vi "fastseq_set_slot-all.vi"(8 "slot":T2 {"slot#" max=4095; "DAC"."DAC offset" min=-1 max=0.5; "DAC"."FastChanNum" max=15 step=1}, 10 "slot number":u16, 11 "FPGA VI Reference In":T1) -> (3 "FPGA VI Reference Out":T1)   [LabVIEW 2013]
uses:
  fpga-bitfile-ref.ctl
  sequence slot/data.ctl
  sequence slot/slot-use.ctl
  sequence slot/triggers.ctl
  sequence slot/DAC.ctl
  sequence slot/DAC_fastseq-offset.ctl
  sequence slot/timing.ctl
  sequence slot/jump.ctl
  sequence slot/slot.xctl
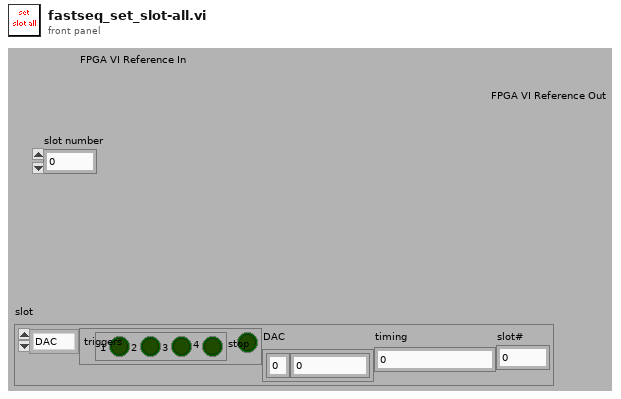
[diagram p1: front panel]
types:
  T1 = typedef "fpga-bitfile-ref.ctl" = refnum<k20>
  T2 = typedef "slot.xctl/data.ctl" = cluster{"use":T3, "Triggers":T4, "DAC":T5, "timing":T7, "slot#":T8}
  T3 = typedef "slot-use.ctl" = enum8{"DAC", "timing", "triggers", "jump"}
  T4 = typedef "triggers.ctl" = cluster{"triggers":cluster{"1":bool, "2":bool, "3":bool, "4":bool}, "stop":bool}
  T5 = typedef "DAC.ctl" = cluster{"FastChanNum":u8, "DAC offset":T6}
  T6 = typedef "DAC_fastseq-offset.ctl" = sgl
  T7 = typedef "timing.ctl" = sgl
  T8 = typedef "jump.ctl" = u16
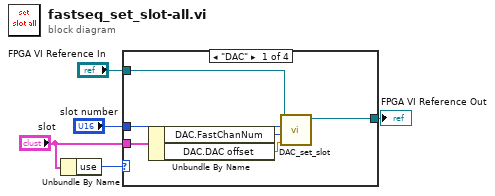
[diagram p0: block diagram]
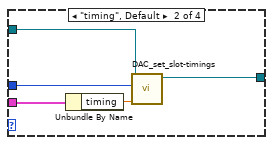
[diagram p2: hidden frame]
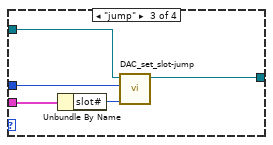
[diagram p3: hidden frame]
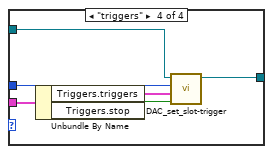
[diagram p4: hidden frame]
diagram:
  n1 = Unbundle By Name("slot") -> ("use"=w3:T3)
  n2 = case shown="\"DAC\"" w3 {
    tunnel: "slot" -> [w11 w16 w21 w27]
    tunnel: "FPGA VI Reference In" -> [w10 w13 w18 w26]
    tunnel: [w9 w12 w19 w25] -> w4
    tunnel: "slot number" -> [w8 w14 w17 w24]
    frame "DAC" {
      n3 = Unbundle By Name(w11) -> ("DAC.FastChanNum"=w7:u8, "DAC.DAC offset"=w6:T6)
      n4 = call "DAC_set_slot.vi"("DAC Offset"=w6, "FastChanNumber"=w7, "slot number"=w8, "FPGA VI Reference In"=w10) -> ("FPGA VI Reference Out"=w9:T1)  [unwired: 7 out]
    }
    frame "timing", Default {
      n5 = Unbundle By Name(w16) -> ("timing"=w15:T7)
      n6 = call "DAC_set_slot-timings.vi"("Time (ms)"=w15, "slot number"=w14, "FPGA VI Reference In"=w13) -> ("FPGA VI Reference Out"=w12:T1)  [unwired: 8 out]
    }
    frame "jump" {
      n7 = Unbundle By Name(w21) -> ("slot#"=w20:T8)
      n8 = call "DAC_set_slot-jump.vi"("JumpTo"=w20, "slot number"=w17, "FPGA VI Reference In"=w18) -> ("FPGA VI Reference Out"=w19:T1)  [unwired: 8 out]
    }
    frame "triggers" {
      n9 = Unbundle By Name(w27) -> ("Triggers.triggers"=w23:cluster{"1":bool, "2":bool, "3":bool, "4":bool}, "Triggers.stop"=w22:bool)
      n10 = call "DAC_set_slot-trigger.vi"("Stop"=w22, "Cluster"=w23, "slot number"=w24, "FPGA VI Reference In"=w26) -> ("FPGA VI Reference Out"=w25:T1)  [unwired: 7 out]
    }
  }
  "FPGA VI Reference Out" <- w4
